vi "lab 2,6,5 ikisi bi,r.vi"() -> ()   [LabVIEW 2020]
uses:
  <vilib>/express/express analysis/Spectral/Block/exnSpectralBlock spectral measurements peak poly.vi
  <vilib>/express/express analysis/Spectral/Block/exnSpectralBlock spectral measurements peak DDT.vi
  <vilib>/express/express analysis/Spectral/XNode/ExpressSpectralMeasurementsBlockNode.xnode
panel:
  in  "rate":dbl=10000.0
  in  "number of samples":i32=993
  out "leakage":dbl
  out "freq":dbl
  out "max value":dbl
  out "resolution":dbl
  out "scallop lose":dbl
  out "amp":dynamicdata(graph)
  out "fft":dynamicdata(graph)
  out "signal":dynamicdata(graph)
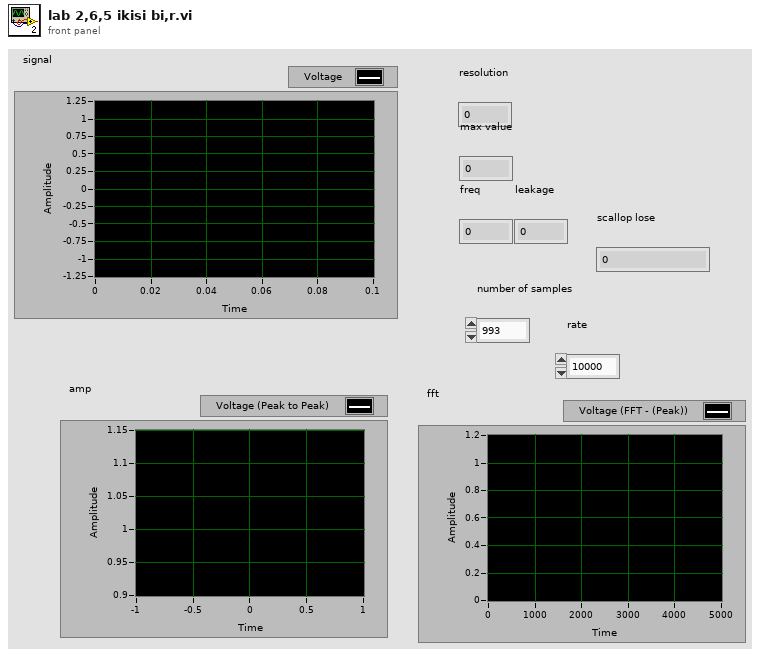
[diagram p1: front panel]
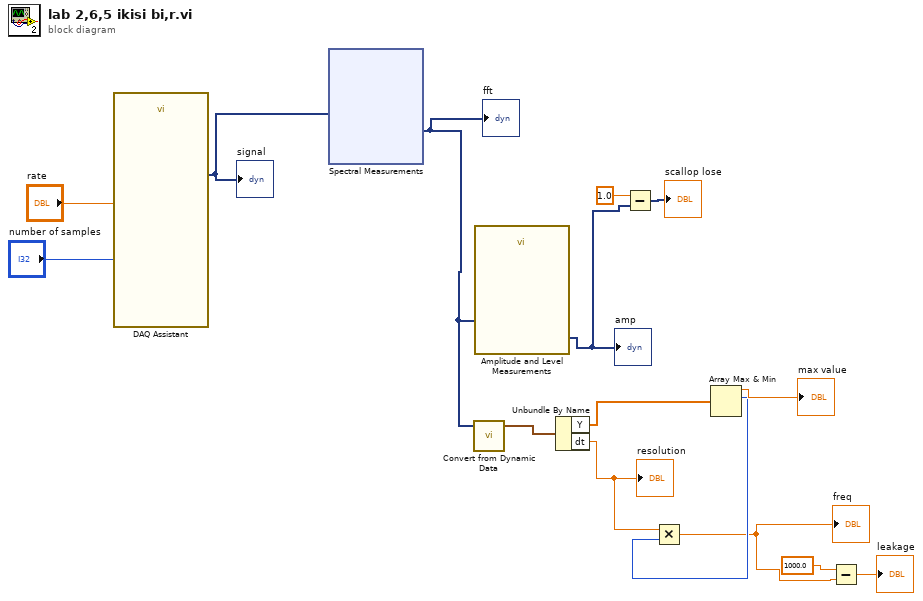
[diagram p0: block diagram]
diagram:
  n1 = call "DAQ Assistant"("rate"="rate", "number of samples"="number of samples") -> ("data"=w15:dynamicdata)  [unwired: 15 in, 2 out]
  "signal" <- w15
  n2 = xnode "Spectral Measurements"("Signals"=w15) -> ("FFT - (Peak)"=w10:dynamicdata)  [unwired: 1 in, 2 out]
  "fft" <- w10
  n3 = call "Convert from Dynamic Data"("Dynamic Data Type"=w10) -> ("Waveform"=w11:waveform(dbl))  [unwired: 3 in]
  n4 = call "Amplitude and Level Measurements"("Signals"=w10) -> ("Peak to Peak"=w13:dynamicdata)  [unwired: 13 in, 1 out]
  "amp" <- w13
  n5 = Unbundle By Name(w11) -> ("Y"=w9:dbl[], "dt"=w6:dbl)
  "resolution" <- w6
  n6 = Subtract(x=1.0, y=w13) -> (x-y=→"scallop lose":dynamicdata)
  n7 = Array Max & Min(array=w9) -> (max value=→"max value":dbl, max index (indices)=w7:i32)  [unwired: 2 out]
  n8 = Multiply(x=w6, y=w7) -> (x*y=w4:dbl)
  "freq" <- w4
  n9 = Subtract(x=1000.0 ("y"), y=w4) -> (x-y=→"leakage":dbl)
